vi "Autotest_Instr.vi"(8 "error in (no error)":errorcluster caption="entrée d'erreur (pas d'erreur)", 11 "Class DIO en entrée":refnum<class "Class Instrument Ana.lvclass">) -> (0 "error out":errorcluster caption="sortie d'erreur", 3 "Class DIO en Sortie":refnum<class "Class Instrument Ana.lvclass">)   [LabVIEW 2020, in "Library Instrument & Equipement.lvlib" / "Library Instruments.lvlib" / "Class Instrument Ana.lvclass"]
uses:
  Class Instrument Ana.lvclass
  C:/Users/ngarcin/OneDrive - Altyor/Standard TB/Class/Instrument/Instrument (Default)/Class Instrument (Default).lvclass
  Class Instrument Ana.lvclass/Class Instrument Ana.ctl
  Instrument (Default)/Class Instrument (Default).lvclass
  Ana/Class Ana (Default)/Class Ana (Default).lvclass
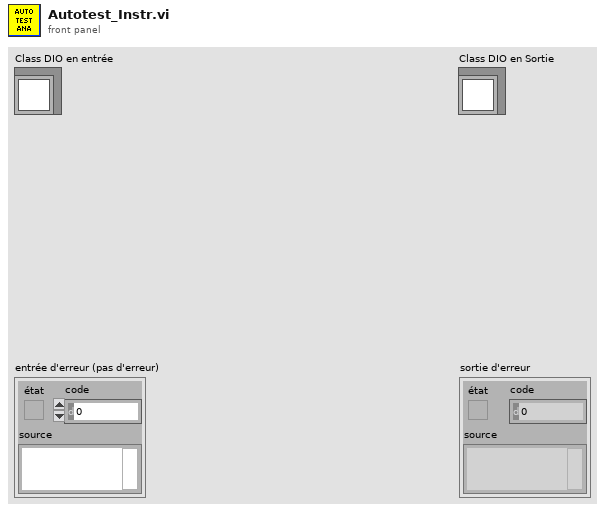
[diagram p1: front panel]
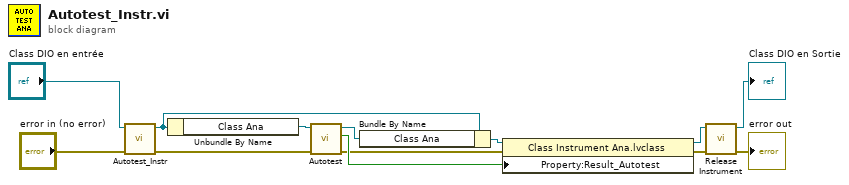
[diagram p0: block diagram]
diagram:
  n1 = call-parent "Autotest_Instr.vi"("error in (no error)"="error in (no error)", "Class Instrument (Default) en entrée"="Class DIO en entrée") -> ("error out"=w2:errorcluster, "Class Instrument (Default) en sortie"=w11:refnum<class "Class Instrument Ana.lvclass">)  [unwired: 8 in]
  n2 = Unbundle By Name(w11) -> ("Class Ana"=w5:refnum<class "Class Ana (Default).lvclass">)
  n3 = call-dynamic "Autotest.vi"("error in (no error)"=w2, "Class DIO (Default) en entrée"=w5) -> ("error out"=w1:errorcluster, "Autotest Ok"=w3:bool, "Class DIO (Default) en sortie"=w4:refnum<class "Class Ana (Default).lvclass">)  [unwired: 7 in]
  n4 = Bundle By Name(cluster=w11, "Class Ana"=w4) -> (w10:refnum<class "Class Instrument Ana.lvclass">)
  n5 = property class="Class Instrument Ana.lvclass"(reference=w10, error in=w1, "Property:Result_Autotest"=w3) -> (reference out=w7:refnum<class "Class Instrument Ana.lvclass">, error out=w9:errorcluster)
  n6 = call-dynamic "Release Instrument.vi"("error in (no error)"=w9, "Class Instrument (Default) en entrée"=w7) -> ("error out"=→"error out":errorcluster, "Class Instrument (Default) en sortie"=→"Class DIO en Sortie":refnum<class "Class Instrument Ana.lvclass">)  [unwired: 8 in]
